vi "SaveGestures.vi"(8 "Error In":errorcluster, 11 ".NET Refnum in":refnum<k24>) -> (0 "Error Out":errorcluster, 3 "All Gestures":T1)   [LabVIEW 2014, in "LMH-Leap.lvlib"]
uses:
  LMH-Leap.lvlib
  C:/github/makerhub/Leap/LabVIEW/vi.lib/LabVIEW Hacker/Leap/Private/Libs/LeapCSharp.NET3.5.dll
  LabVIEW Hacker/Leap/Private/Libs/LeapCSharp.NET3.5.dll
  Type Defs/All Gestures.ctl
  Type Defs/Gesture Swipe.ctl
  Type Defs/Gesture Common.ctl
  Type Defs/Gesture Type.ctl
  Type Defs/Gesture State.ctl
  Type Defs/Vector.ctl
  Type Defs/Gesture Circle.ctl
  Type Defs/Gesture Screen Tap.ctl
  Type Defs/Gesture Key Tap.ctl
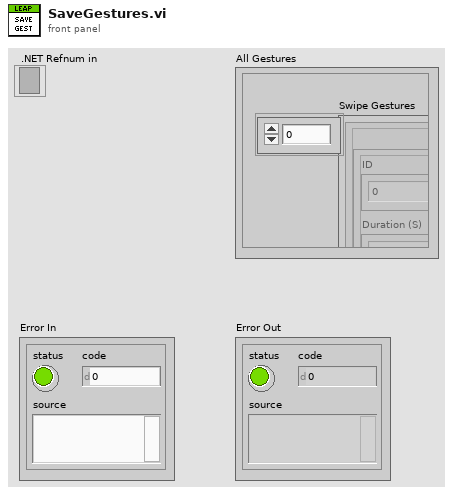
[diagram p1: front panel]
types:
  T1 = typedef "LMH-Leap.lvlib/All Gestures.ctl" = cluster{"Swipe Gestures":T2[], "Circle Gestures":T7[], "Screen Tap Gestures":T8[], "Key Tap Gestures":T9[]}
  T2 = typedef "LMH-Leap.lvlib/Gesture Swipe.ctl" = cluster{"Common":T3, "Direction":T6, "Position":T6, "Start Position":T6, "Speed":dbl}
  T3 = typedef "LMH-Leap.lvlib/Gesture Common.ctl" = cluster{"ID":dbl, "Duration (S)":dbl, "Gesture Type":T4, "Gesture State":T5}
  T4 = typedef "LMH-Leap.lvlib/Gesture Type.ctl" = enum16{"Invalid", "Swipe", "Circle", "Screen Tap", "Key Tap"}
  T5 = typedef "LMH-Leap.lvlib/Gesture State.ctl" = enum16{"Invalid", "Start", "Update", "Stop"}
  T6 = typedef "LMH-Leap.lvlib/Vector.ctl" = cluster{"Pitch":sgl, "Yaw":sgl, "Roll":sgl, "Magnitude":sgl, "XYZ":sgl[]}
  T7 = typedef "LMH-Leap.lvlib/Gesture Circle.ctl" = cluster{"Common":T3, "Center":T6, "Normal":T6, "Progress":dbl, "Radius":dbl}
  T8 = typedef "LMH-Leap.lvlib/Gesture Screen Tap.ctl" = cluster{"Common":T3, "Direction":T6, "Position":T6, "Progress":dbl}
  T9 = typedef "LMH-Leap.lvlib/Gesture Key Tap.ctl" = cluster{"Common":T3, "Direction":T6, "Position":T6, "Progress":dbl}
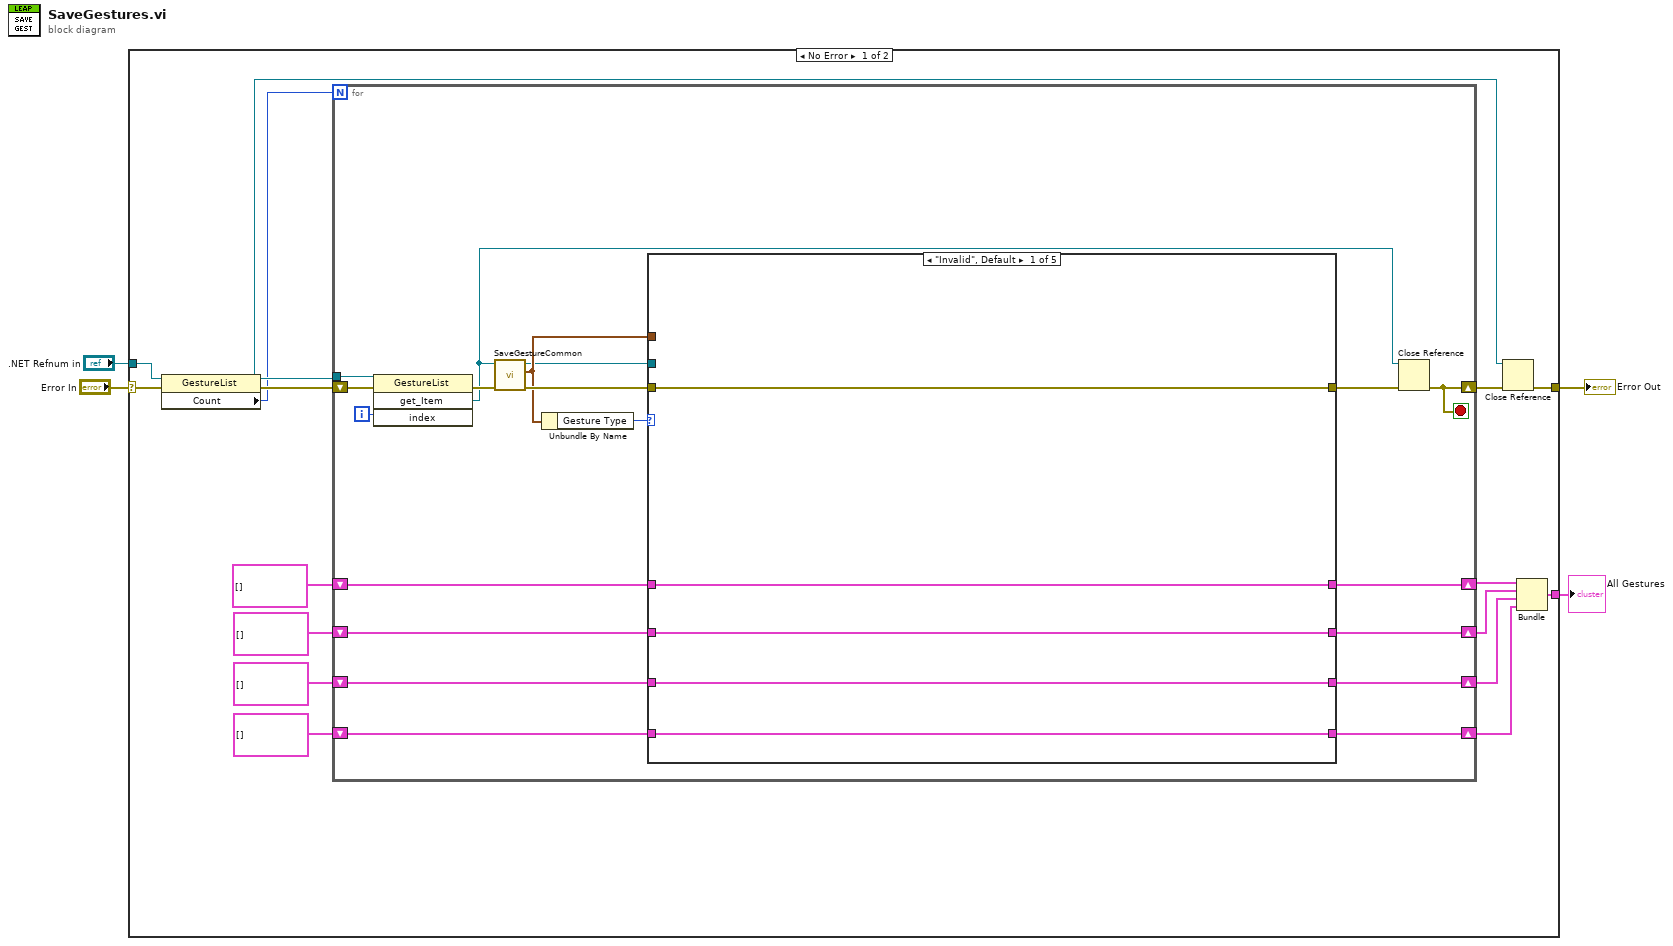
[diagram p0: block diagram]
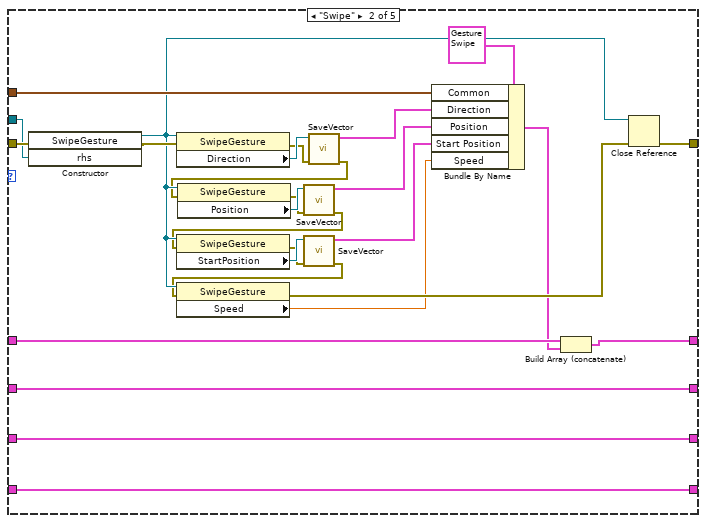
[diagram p2: hidden frame]
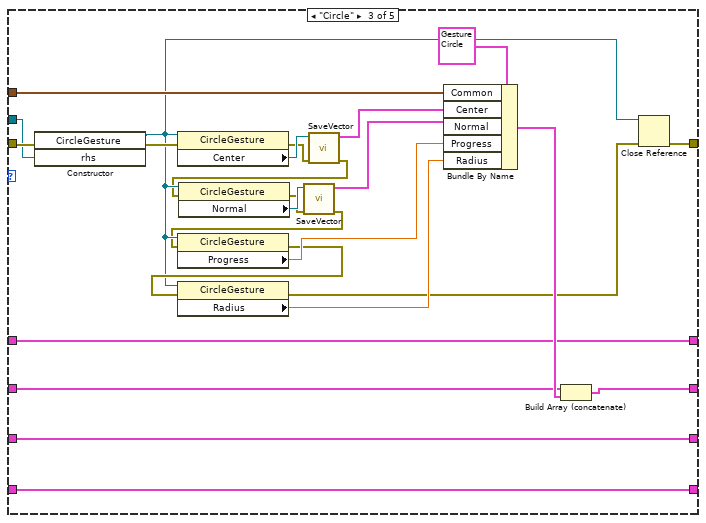
[diagram p3: hidden frame]
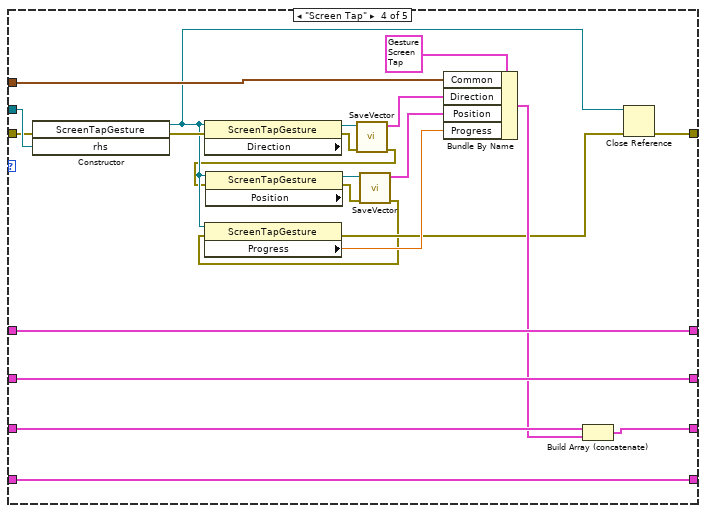
[diagram p4: hidden frame]
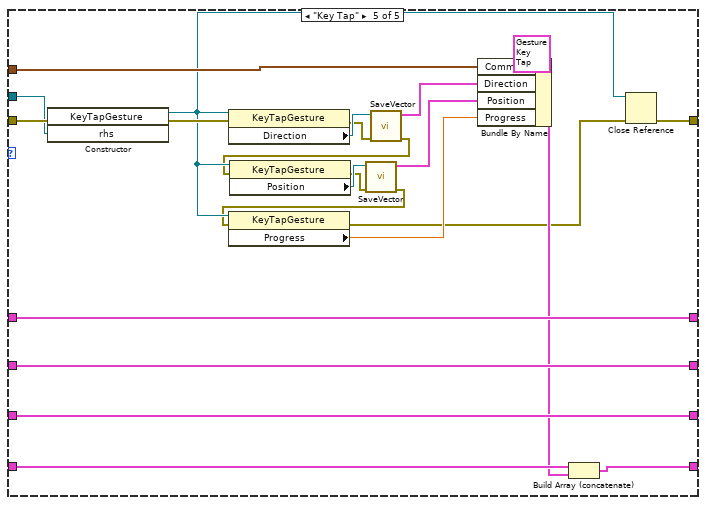
[diagram p5: hidden frame]
diagram:
  n1 = case shown="No Error" "Error In" {
    selector: "Error In" -> [w17 w143]
    tunnel: ".NET Refnum in" -> [w18 _]
    tunnel: [w15 w143] -> w2
    tunnel: [w5 _] -> w3
    frame No Error {
      n2 = property class="GestureList"(reference=w18, error in=w17) -> (reference out=w19:refnum<k24>, error out=w20:errorcluster, "Count"=w14:i32)
      n3 = for {
        N: w14 -> [_]
        tunnel: w19 -> [w37]
        shift-right: [w35] -> w16
        shift-left: w20 -> [w38]
        shift-right: [w29] -> w9
        shift-left: T2[] [] -> [w30]
        shift-right: [w27] -> w8
        shift-left: T7[] [] -> [w28]
        shift-right: [w25] -> w7
        shift-left: T8[] [] -> [w26]
        shift-right: [w23] -> w6
        shift-left: T9[] [] -> [w24]
        i -> [w36]
        stop <- w35 stop-if-true
        n4 = invoke class="GestureList" method="get_Item"(reference=w37, error in=w38, "index"=w36) -> (error out=w39:errorcluster, "get_Item"=w22:refnum<k24>)  [unwired: 1 in, 2 out]
        n5 = call "SaveGestureCommon.vi"("Error In"=w39, ".NET Refnum in"=w22) -> ("Error Out"=w34:errorcluster, "Gesture Common"=w31:T3, ".NET Refnum Passthrough"=w21:refnum<k24>)  [unwired: 7 in]
        n6 = Unbundle By Name(w31) -> ("Gesture Type"=w33:T4)
        n7 = case shown="\"Invalid\", Default" w33 {
          tunnel: w21 -> [_ w53 w80 w106 w124]
          tunnel: w34 -> [w44 w55 w81 w105 w129]
          tunnel: [w44 w52 w78 w103 w127] -> w32
          tunnel: w31 -> [_ w69 w96 w119 w142]
          tunnel: w30 -> [w43 w61 w84 w113 w136]
          tunnel: [w43 w59 w84 w113 w136] -> w29
          tunnel: w28 -> [w42 w58 w86 w111 w135]
          tunnel: [w42 w58 w85 w111 w135] -> w27
          tunnel: w26 -> [w41 w57 w83 w110 w134]
          tunnel: [w41 w57 w83 w108 w134] -> w25
          tunnel: w24 -> [w40 w56 w82 w107 w132]
          tunnel: [w40 w56 w82 w107 w130] -> w23
          frame "Invalid", Default {
          }
          frame "Swipe" {
            n8 = constructor class="SwipeGesture"(error in=w55, "rhs"=w53) -> (reference out=w51:refnum<k24>, error out=w54:errorcluster)  [unwired: 2 in, 2 out]
            n9 = property class="SwipeGesture"(reference=w51, error in=w54) -> (error out=w50:errorcluster, "Direction"=w68:refnum<k24>)  [unwired: 1 out]
            n10 = call "SaveVector.vi"("error in (no error)"=w50, "Leap Vector"=w68) -> ("error out"=w49:errorcluster, "Vector"=w65:T6)  [unwired: 8 in]
            n11 = property class="SwipeGesture"(reference=w51, error in=w49) -> (error out=w48:errorcluster, "Position"=w67:refnum<k24>)  [unwired: 1 out]
            n12 = call "SaveVector.vi"("error in (no error)"=w48, "Leap Vector"=w67) -> ("error out"=w47:errorcluster, "Vector"=w64:T6)  [unwired: 8 in]
            n13 = property class="SwipeGesture"(reference=w51, error in=w47) -> (error out=w46:errorcluster, "StartPosition"=w66:refnum<k24>)  [unwired: 1 out]
            n14 = call "SaveVector.vi"("error in (no error)"=w46, "Leap Vector"=w66) -> ("error out"=w45:errorcluster, "Vector"=w63:T6)  [unwired: 8 in]
            n15 = property class="SwipeGesture"(reference=w51, error in=w45) -> (error out=w71:errorcluster, "Speed"=w62:sgl)  [unwired: 1 out]
            n16 = Bundle By Name(cluster=T2 {"Common"={"ID"=0.0, "Duration (S)"=0.0, "Gesture Type"=enum."Invalid", "Gesture State"=enum."Invalid"}, "Direction"={"Pitch"=nan, "Yaw"=nan, "Roll"=nan, "Magnitude"=nan, "XYZ"=[nan, nan, nan]}, "Position"={"Pitch"=nan, "Yaw"=nan, "Roll"=nan, "Magnitude"=nan, "XYZ"=[nan, nan, nan]}, "Start Position"={"Pitch"=nan, "Yaw"=nan, "Roll"=nan, "Magnitude"=nan, "XYZ"=[nan, nan, nan]}, "Speed"=0.0} ("Gesture Swipe"), "Common"=w69, "Direction"=w65, "Position"=w64, "Start Position"=w63, "Speed"=w62) -> (w60:T2)
            n17 = Build Array (concatenate)(w61, w60) -> (w59:T2[])
            n18 = Close Reference(reference=w51, error in (no error)=w71) -> (error out=w52:errorcluster)
          }
          frame "Circle" {
            n19 = constructor class="CircleGesture"(error in=w81, "rhs"=w80) -> (reference out=w76:refnum<k24>, error out=w79:errorcluster)  [unwired: 2 in, 2 out]
            n20 = property class="CircleGesture"(reference=w76, error in=w79) -> (error out=w75:errorcluster, "Center"=w95:refnum<k24>)  [unwired: 1 out]
            n21 = call "SaveVector.vi"("error in (no error)"=w75, "Leap Vector"=w95) -> ("error out"=w74:errorcluster, "Vector"=w93:T6)  [unwired: 8 in]
            n22 = property class="CircleGesture"(reference=w76, error in=w74) -> (error out=w73:errorcluster, "Normal"=w94:refnum<k24>)  [unwired: 1 out]
            n23 = call "SaveVector.vi"("error in (no error)"=w73, "Leap Vector"=w94) -> ("error out"=w72:errorcluster, "Vector"=w92:T6)  [unwired: 8 in]
            n24 = property class="CircleGesture"(reference=w76, error in=w72) -> (error out=w87:errorcluster, "Progress"=w88:sgl)  [unwired: 1 out]
            n25 = property class="CircleGesture"(reference=w76, error in=w87) -> (error out=w77:errorcluster, "Radius"=w91:sgl)  [unwired: 1 out]
            n26 = Bundle By Name(cluster=T7 {"Common"={"ID"=0.0, "Duration (S)"=0.0, "Gesture Type"=enum."Invalid", "Gesture State"=enum."Invalid"}, "Center"={"Pitch"=nan, "Yaw"=nan, "Roll"=nan, "Magnitude"=nan, "XYZ"=[nan, nan, nan]}, "Normal"={"Pitch"=nan, "Yaw"=nan, "Roll"=nan, "Magnitude"=nan, "XYZ"=[nan, nan, nan]}, "Progress"=0.0, "Radius"=0.0} ("Gesture Circle"), "Common"=w96, "Center"=w93, "Normal"=w92, "Progress"=w88, "Radius"=w91) -> (w90:T7)
            n27 = Build Array (concatenate)(w86, w90) -> (w85:T7[])
            n28 = Close Reference(reference=w76, error in (no error)=w77) -> (error out=w78:errorcluster)
          }
          frame "Screen Tap" {
            n29 = constructor class="ScreenTapGesture"(error in=w105, "rhs"=w106) -> (reference out=w101:refnum<k24>, error out=w104:errorcluster)  [unwired: 2 in, 2 out]
            n30 = property class="ScreenTapGesture"(reference=w101, error in=w104) -> (error out=w100:errorcluster, "Direction"=w118:refnum<k24>)  [unwired: 1 out]
            n31 = call "SaveVector.vi"("error in (no error)"=w100, "Leap Vector"=w118) -> ("error out"=w99:errorcluster, "Vector"=w116:T6)  [unwired: 8 in]
            n32 = property class="ScreenTapGesture"(reference=w101, error in=w99) -> (error out=w98:errorcluster, "Position"=w117:refnum<k24>)  [unwired: 1 out]
            n33 = call "SaveVector.vi"("error in (no error)"=w98, "Leap Vector"=w117) -> ("error out"=w97:errorcluster, "Vector"=w115:T6)  [unwired: 8 in]
            n34 = property class="ScreenTapGesture"(reference=w101, error in=w97) -> (error out=w102:errorcluster, "Progress"=w114:sgl)  [unwired: 1 out]
            n35 = Bundle By Name(cluster=T8 {"Common"={"ID"=0.0, "Duration (S)"=0.0, "Gesture Type"=enum."Invalid", "Gesture State"=enum."Invalid"}, "Direction"={"Pitch"=nan, "Yaw"=nan, "Roll"=nan, "Magnitude"=nan, "XYZ"=[nan, nan, nan]}, "Position"={"Pitch"=nan, "Yaw"=nan, "Roll"=nan, "Magnitude"=nan, "XYZ"=[nan, nan, nan]}, "Progress"=0.0} ("Gesture Screen Tap"), "Common"=w119, "Direction"=w116, "Position"=w115, "Progress"=w114) -> (w109:T8)
            n36 = Build Array (concatenate)(w110, w109) -> (w108:T8[])
            n37 = Close Reference(reference=w101, error in (no error)=w102) -> (error out=w103:errorcluster)
          }
          frame "Key Tap" {
            n38 = constructor class="KeyTapGesture"(error in=w129, "rhs"=w124) -> (reference out=w125:refnum<k24>, error out=w128:errorcluster)  [unwired: 2 in, 2 out]
            n39 = property class="KeyTapGesture"(reference=w125, error in=w128) -> (error out=w123:errorcluster, "Direction"=w141:refnum<k24>)  [unwired: 1 out]
            n40 = call "SaveVector.vi"("error in (no error)"=w123, "Leap Vector"=w141) -> ("error out"=w122:errorcluster, "Vector"=w139:T6)  [unwired: 8 in]
            n41 = property class="KeyTapGesture"(reference=w125, error in=w122) -> (error out=w121:errorcluster, "Position"=w140:refnum<k24>)  [unwired: 1 out]
            n42 = call "SaveVector.vi"("error in (no error)"=w121, "Leap Vector"=w140) -> ("error out"=w120:errorcluster, "Vector"=w138:T6)  [unwired: 8 in]
            n43 = property class="KeyTapGesture"(reference=w125, error in=w120) -> (error out=w126:errorcluster, "Progress"=w137:sgl)  [unwired: 1 out]
            n44 = Bundle By Name(cluster=T9 {"Common"={"ID"=0.0, "Duration (S)"=0.0, "Gesture Type"=enum."Invalid", "Gesture State"=enum."Invalid"}, "Direction"={"Pitch"=nan, "Yaw"=nan, "Roll"=nan, "Magnitude"=nan, "XYZ"=[nan, nan, nan]}, "Position"={"Pitch"=nan, "Yaw"=nan, "Roll"=nan, "Magnitude"=nan, "XYZ"=[nan, nan, nan]}, "Progress"=0.0} ("Gesture Key Tap"), "Common"=w142, "Direction"=w139, "Position"=w138, "Progress"=w137) -> (w131:T9)
            n45 = Build Array (concatenate)(w132, w131) -> (w130:T9[])
            n46 = Close Reference(reference=w125, error in (no error)=w126) -> (error out=w127:errorcluster)
          }
        }
        n47 = Close Reference(reference=w22, error in (no error)=w32) -> (error out=w35:errorcluster)
      }
      n48 = Close Reference(reference=w19, error in (no error)=w16) -> (error out=w15:errorcluster)
      n49 = Bundle(w9, w8, w7, w6) -> (w5:cluster{T2[], T7[], T8[], T9[]})  [unwired: 1 in]
    }
    frame Error {
    }
  }
  "All Gestures" <- w3
  "Error Out" <- w2
